vi "Day 20-1.vi"() -> ()   [LabVIEW 2020]
uses:
  Vec2.ctl
panel:
  out "# Lit":i32
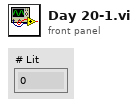
[diagram p1: front panel]
types:
  T1 = typedef "Vec2.ctl" = cluster{"X":i32, "Y":i32}
  T2 = typedef "Puzzle 20-1.ctl" = cluster{"Enhancement":bool[], "Image":map{T1, bool}, "Fill":bool, "Min":T1, "Max":T1}
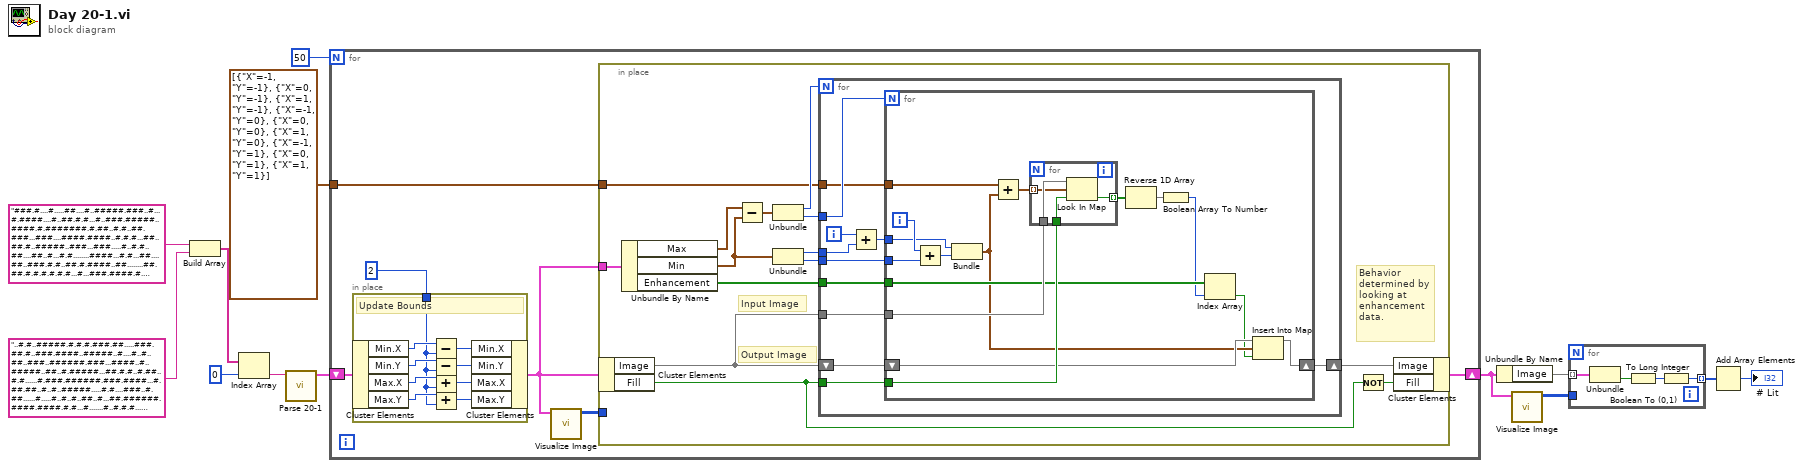
[diagram p0: block diagram]
diagram:
  n1 = Build Array("###.#....#.....##....#..#####.###..#...#.####....#..##.#.#...#..###.#####..####.#.#######.#.##..#.#..##.###...###....####.####..#.#.#...##..##.#..#####..###...###.....#..#.#..##....##..#...#.#........####...#.#...##....##..###.#.#..##.#.####..##........##.##.#.#.#.#.#.#...#...###.####.#.######..#.#.##....#.##.....##.#.#.#.##...#...#.#..#..##.#######.###............####...###.#..#.###.#...#.......#.##.##...##..####.##....#####....#..#...#.#.##.#......#####....#####..#..#.##...#.#....##.##..###....##.#....##.\n\n.......#............#.##...##..#...##.#..####.#..#.##..#.##.##..#.#....#.#####.#.##..#..#..##..#.###\n.#.####.......#....##....#####.##...######.###.##....####..####.#....#..####..#....#.##..##.##..##..\n.###.##.#.##.#......#...##.#.#.##..##..##....##...#####...#####..###......####...###.#.###.##.##.##.\n###.##.....###.##...###..#..##.#.#....####..###.###..###..###.#..#..#..##...#....##..#..####..#...#.\n..#######..#...##..####.#.#.#.##.#.##.######..#.##.#..####.#.##.####.#.#..##.#.....#.#...###.###....\n#.###.#....#.###..#.....##....#..##.....#####..###.#..#.####..#....#......#.#.##.#...#####..#.#.####\n.###.##.##.##..#...#.#.###.#.#####.########.....#####.#.......##...##....#.#.###...#..#...##.#.#.#..\n.###..###....###.###.###.##.###...##.##.....####.#.##.##..#####.#.#.##..##....##.#..#.#..#..#..#.#..\n###.#.....#.##.#..#...###.###..##..##...##..#.#.####.#.###.##.#.###..##..#.##.#.#.#..#####..#.#.#..#\n###.#....#.#...######.##..#.####..##.....#.###.....###...##....###.#######..#......#....####.#..#..#\n..#...#...#.##.#....###.#######....###..###.#####.###.#..#.....#.#.###.#...#.###..##.#.#.##.##.##...\n##...#.....##.#.##.##..#..#...#........##....#.#.#....#..##..####..#....#####.##.##..###.###.####.##\n.#.###.....#...##...#..#..###..#.##..#.##..##.#.##.#.##.#.###...####.#.#...##...####.#....#.#....#.#\n########.#.#.#.....##.##..###.#..#.#####.##.##.##.##.#..#..#.#.###.##########..##...#..###..#.##..#.\n......##.##..##.###.####...###.#..##.#.##.####.####...#######..#..#.###..##...###.###.#.#.#.######.#\n.###.####.#####.#.#.#...##.#.##....#..##.#####.####....#.....##.#.#..##....##..#.#.####...#.##...#.#\n##....######...#..##..#.#####.##.#####..#......#.#.#..#######.#...##.##..##..#..#.###.#.#......##.#.\n.##......#..#...#..##..#.#.###..##.#..###.###.##.##.#...#.#.##.#.###....#####....##...##...####.###.\n####.###....###..###.###......####.#..#####.#......##....#...##..#####....#.#######.##...##.##.##.##\n#....##.####....#####...##......####.#.#.#.##....#.###.#...##.##...#.#.##.#....#..#.##.#.#..#.#..##.\n#.##.#.##..##.#.##...#####.###.#..##.....###...#.##.###....#.###..###.####....###..##.###.#..######.\n..#...##...#...#...#..###..#..#.#......##.#...#...#..#.#..#..#.##.#####...#..##..###...#.###..#....#\n.##...#.#.....#.###...###....#####...##.#.###..##..###.#...######.#####.#..####.#....###.####..#...#\n#.##.##.#.#.#..#.#####.###.###.#.###..#.#.##..####.#.######.#.###.#.##...#..#..#..#.#.#..#.#.#..##..\n#####.####.##.#..##.......#....#...#.#.....#..#.#...#.......##.#######.#.##....#.....##...##...###.#\n##.#...#.#..####.##.###.####..###..###..#...#.######.##.##.#.#.#..###.#.##.#.#.#..#####..###.##....#\n.#.##.#.#......#......###.#.####..#.#..###....#####..###..#.######....##..##.##.##....#..#........#.\n.##.##..#####.....#.###.....#.##....#.....#.#.#..#..#######..#####.....##.###.###.##..##..###...##.#\n#..#.#.#.####..###.#.##.......#.#.#.#.##.#.#.#.#..##.##.##.......#.#.#..#..###...#.##.#.#..#....###.\n.#####.#.##.#..#.#...####...###.####.#.#.....####..#...#.###...#....#.#..####.####...#....#.##.###..\n.....##..#.##.#######....###...##...#.#.##.#..###....#.##..###....##..##.#.###.##..#####........#.##\n##.#.#.#########..##....#..#.##.#...#..#....##..#.###.#.#.#.###.#.....#......##.##....#.....#.#...##\n..##..#..#.##...#.....##.##....##.####....#...###..##...##.#......#...#.....#....##...###.###....#..\n##.#.##.....#.#.##..#......#...####....#.##.#.##..####.##.#.###.#...#..#..##..###..#.###.####.####.#\n.#.#..####.##.#.###..##.#.###..##.##..#...##..#..#.##..####..####..#...###.######....###.#..#####..#\n#.##..##.##...#....##...###..#.##...##....#.....#..##.#.###....#......##.##..###.#..######....##.#..\n#.####.....##.###.##...###.###.#....#.....####.#####......#.#......#..##...##.#....###.##.#....#..#.\n...###..###.#.#.###.#.#.##.####.#.######.#.##..#...#..##.#.#.#.#.............#..#.#.###.....##.###..\n#...###.#.##.####..##...###.##...####.##....######.....######.##.##.#..#.##.##.#......#.###.#.#...##\n####.#.########.##...##.############...###.##...#...######....##.########.##.##..#...##..#.#...##.##\n###.#..#..##.##....#..#..#..##.#.##.##.......##..#...#.###.#.#....##.#.#.##.#####.##.......#.#.#..##\n..#######.####.##...#####.#.####.#...#...#..#..##.###.#########....#..###.##..#.##..##.....###.#..#.\n###.#.#..#.#..###.#.#..#.##...##....#.#..#.......#.###.#.#.#.#####...#...######.##.#....##.#..#.#.#.\n.##....#.#.###...#.#...####..###.#.#.#..##.##.#..##...#...####..#......#####..####..##.##.##...##..#\n...##.##..#.#.....##...#..##.#.#.####..##.........##..##.....#.###.##...##.##..#..#...#..#......####\n......#..#####.....#....##..#####...#.#.##......##....####...#...####.###.#.#.##..#..#...##...###...\n...###....###.####.#....###......#.#...#.##.#..#######..#....#####.##.#####..###....##.##..##....#.#\n##...###.####..#...#.##....#..#.#.#..#.#....#.#...#.##..#..######.....##..#.#.######.#.#....##.#.#.#\n#..##...#..#.##.....####.##.##.#.#.##.#..##..##..#...#####.###.###........#.#.#..#.#.##.#...##..#.#.\n#####..##....#.#..##.#.##..#.###..##..#.#.###.####.#.#..#.....#..##.####..#.####.###..#.....##....##\n.##..###.#.#.#.#.####.#.##...###..#####.####.###.##.###.##.#....#.#.#..#.#.##.#..####...###.####.##.\n#.#.#......#.###.#...###..###...#...#.#..######.###.##.#.####.....#...##.#..##..##.#..##.#.#....#.##\n#...##...##.#...##....######.########....#..#######.#.####....#..##..##.##.#.###.####.####..###.####\n#.##..##...#.####.#.#..####.#.##.#.#...####...####.#.#....####..##...#......#........##........####.\n..##.#..######...#####.#.##.###.##.......#..###..###...#....#..####..#..#..#...##.#.##.####.#.##.#..\n#..#...###..#..#.#...###.#..#.#...#.....##..#.#...#####...##....##.......####.##..####..##.#..######\n.##.####..###..##.#.####.###.##...##..###.#.#.##...##.....#..#..#.####..###...##...#######.....##.#.\n.####.#.#.##...##...###.....####.##..####....##....#...##.##...##.####.###.##...#####..#...#.#...#..\n....#.#...#..#.#.#....####.##..#.#....#........#...####..###..###.###...#..###.#..#.##.#..#...#.####\n#..#..##..##.#...#####...#.......#..##..###.#.#.####..###.#...##......##.##.#..#.#.##.#..##.#.#...#.\n.#####...#.##.###.#.##..###.##.#.#...##..#.#...###.....##.#.##.#..#..####...#.######....#..#.##..#..\n#.#...#.....#.....######.##.##.##.##.#.#..#..#.#.####..#...#####.##.####..###.##.#.#.#.#..#.#...####\n##.##.#.#...##.#.###.#####.#...##.........#......#.##.....#.......##....#.#.##..#.#..#.#..##..#.###.\n....#.#.##.###.##..##.#..#.##.#..#.######.###.##..#..#.#...###.#........###.###.##..####.#...###..#.\n#####..####.#.###..#####...#.......#.##.#.....#.###.####.......##.#.#.##.#...#....#....#....##...##.\n.##.#..####...##...##.....##..#.####.#...#..##..#....####.#..#..#.#..#...#.#.#.##.####..######..#.#.\n#.#.##.##.#.....#...#..#...#.#.#..#.#.#####..#.##..#.##.#......##.#..#.#.#...#...####.#.#.#.#....#..\n.##..###.##..##...#..##...#..#......#.#####.####.####.#.......##.#.#..#..#.#.##.#..#..###.#.#..##..#\n#..##...#........##..#...###########.#.###...##.##...##.#.###...####..########..#...##..####..###...\n.#.#..###.#.##.#.#..#######......####.#....#####...##...#.###.##....#####.#...#######.######..######\n.#.###..###.##...#...###.########...#.#.#.#..#...#..#.#.....####..#...####......#.#...##.#.###..##.#\n#.###.###...#..#####.###.#...###..#..#..###.#..#..###.#..##.####..#####..#....#....##.##.#..#.####.#\n..#.###.#.#.#.#...####.#.##.#...#.##...#.###.##.#.#######.#####.##..####....###.###.##.#.##....##.##\n#..#.....#..#.##.#....#.####..#.##..####.#..#.#.###..##..#..#..##.####........#..#....#.#.#.###.##..\n#.##.#.#..##.#####...##.#...#..#...#.#.##.#..##.....##.##.#.#.#.###......#.###.###..###.###..#######\n##.###.###...#..##.....#######..##.#.##..#.#.....###.#....####.####.#..##.#..#..#..##.....#..###..##\n#....#..#.#.#..#.#....#.##.#.#.#.###.###.###.##..##.####..####.#.#....#.#######..###.#.....####.#..#\n###.....#.#####..###.#.#....#.....#.###....##..###.#..#.#.#...###.##....#....#..#......#..#....#..#.\n.#.#.#.#####........#.#######...#.####...#...#.###..#....#.#.###.##.....##.#.##..#.#.....#.#..##..##\n...###..#....#.###.#.#.#..##.##.....##.##...#.#........#.#.#####.#...####.#...##..##......#####.###.\n##.###..#.#...#......#######.#..##....###.#.##.#..###.#..###.#...#..######..........##.#.#.#..#..##.\n#..###.#...##..#######..#..#.###..#.###.##.######.##.###.##..#######.#..###.##.##...###....##..#.#.#\n#.#....#..#.###.#.##...#####.##....#...#.##.#..#.##..#...#...##.#..#..#.#.#..#####..##.###....#.#.##\n###...#.#.#..####.....##.#.##.##..#.####...###....###.#.##.########..#####.##.##.#..#....###..###.##\n##.###...#.#.#.#.##...##.#.##.#.#..#.#.#.###.##.#.##.##....########.#..#####..##.#.#.#..#####.#..###\n##..##.##.###.#######.##.......#.#.##.###..##...#...##...#####.#....#.#.#...#.#..#.#.#..####.###.#.#\n###..#.#..#..#..####.#.#.####..#....######...####..######.##.##..#####....####...##########..#####.#\n...#####.#.##....##.##....#...##...##.#.#.#.#.......#.##.#...####.##..####.....#...##..##.#...##...#\n#####.#.###..#..###.#..#..##..##.#.#.#.#..#...###...#.###.###.###..#.#.##.#####...#.#.##.#....#####.\n###.#..###.#.####.#.#..#.##.##.#.#.##......##.####..#...#....##..#....#.#..#..##...###...##.##.#.#..\n..#.#..#...##.#....###.##...#...##.##..###..#.#.#.......##.#.#..#.##.#......#.#..#..#...#...#.#.#.##\n#.#.#.#..###.##.#.#####.###.#.#..###....###...###....#.#..#.......##.#.###..##..#...###.#.##....#..#\n.#..##......#.#.....##.#...##....####....##.####..#....#...##.######.#..#.#.#....#.#######.....####.\n..#..###....##.##..##..#.#..####..##...#.####..........##.#.#.#..##..#..#.##....###.####.....#..##.#\n....#.#.....#.#..#....#..#.###.####..#..##.####....##....#.#..#.#.####.##.......##.##.###.#.##..#.#.\n..###.##....#.##......####..###..#..##.########.###.##...###.#.....#...###.#..#..#.#....#..#.######.\n.##.#.........#..#.#..#.#.##.####.#..##...#.###....#..#...##..##.#..#..####.#...#...####.....##...##\n##..#.#.##.##.#...######..##.##.#.#.#.###..#.#.#....###......##...#.#....#...##.########.##..####.##\n.#......##.###...##..##..###.####.#....##.#.#.#....##.#....##...######.....##..##....#.###..#..#.##.\n#...#...#.......#.#.#####.#..###..#..#...###...###..#.#.......###.#..##.#####...##.#####...#.#.####.", "..#.#..#####.#.#.#.###.##.....###.##.#..###.####..#####..#....#..#..##..###..######.###...####..#..#####..##..#.#####...##.#.#..#.##..#.#......#.###.######.###.####...#.##.##..#..#..#####.....#.#....###..#.##......#.....#..#..#..##..#...##.######.####.####.#.#...#.......#..#.#.#...####.##.#......#..#...##.#.##..#...##.#.##..###.#......#.#.......#.#.#.####.###.##...#.....####.#..#..#.##.#....##..#.####....##...##..#...#......#.#.......#.......##..####..#...#.#.#...##..#.#..###..#####........#..####......#..#\n\n#..#.\n#....\n##..#\n..#..\n..###") -> (w11:string[])
  n2 = Index Array(array=w11, index=0) -> (element=w9:string)
  n3 = call "Parse 20-1.vi"("String"=w9) -> ("Puzzle"=w8:T2)  [unwired: 10 in]
  n4 = for {
    N: 50 -> [_]
    shift-right: [w18] -> w2
    shift-left: w8 -> [w19]
    tunnel: T1[] [{"X"=-1, "Y"=-1}, {"X"=0, "Y"=-1}, {"X"=1, "Y"=-1}, {"X"=-1, "Y"=0}, {"X"=0, "Y"=0}, {"X"=1, "Y"=0}, {"X"=-1, "Y"=1}, {"X"=0, "Y"=1}, {"X"=1, "Y"=1}] -> [w17]
    n5 = in-place {
      in-place-border: 2 -> [w65]
      # "Update Bounds"
      n6 = in-place-cluster #1(w19) -> ("Min.X"=w73:i32, "Min.Y"=w70:i32, "Max.X"=w67:i32, "Max.Y"=w66:i32)
      n7 = Subtract(x=w73, y=w65) -> (x-y=w72:i32)
      n8 = Subtract(x=w70, y=w65) -> (x-y=w71:i32)
      n9 = Add(x=w67, y=w65) -> (x+y=w69:i32)
      n10 = Add(x=w66, y=w65) -> (x+y=w68:i32)
      n11 = in-place-cluster #1("Min.X"=w72, "Min.Y"=w71, "Max.X"=w69, "Max.Y"=w68) -> (w16:T2)
    }
    n12 = call "Visualize Image.vi"("Puzzle 20-1"=w16) -> ("Image"=w15:i16[][])  [unwired: 10 in]
    n13 = in-place {
      in-place-border: w16 -> [w33]
      in-place-border: w17 -> [w22]
      in-place-border: w15 -> [_]
      # "Input Image"
      # "Output Image"
      # "Behavior determined by looking at enhancement data."
      n14 = in-place-cluster #2(w16) -> ("Image"=w20:map{T1, bool}, "Fill"=w21:bool)
      n15 = Unbundle By Name(w33) -> ("Max"=w32:T1, "Min"=w29:T1, "Enhancement"=w25:bool[])
      n16 = Subtract(x=w32, y=w29) -> (x-y=w31:T1)
      n17 = Unbundle(w31) -> ("X"=w30:i32, "Y"=w28:i32)
      n18 = Unbundle(w29) -> ("X"=w27:i32, "Y"=w26:i32)
      n19 = for {
        N: w30 -> [_]
        tunnel: w28 -> [w44]
        tunnel: w27 -> [w43]
        tunnel: w26 -> [w40]
        tunnel: w25 -> [w39]
        shift-right: [w37] -> w24
        shift-left: w20 -> [w38]
        tunnel: w22 -> [w35]
        tunnel: w20 -> [w34]
        tunnel: w21 -> [w36]
        i -> [w42]
        n20 = Add(x=w42, y=w43) -> (x+y=w41:i32)
        n21 = for {
          N: w44 -> [_]
          tunnel: w41 -> [w58]
          tunnel: w40 -> [w60]
          tunnel: w39 -> [w51]
          shift-right: [w46] -> w37
          shift-left: w38 -> [w49]
          tunnel: w35 -> [w56]
          tunnel: w34 -> [w54]
          tunnel: w36 -> [w53]
          i -> [w59]
          n22 = Add(x=w59, y=w60) -> (x+y=w57:i32)
          n23 = Bundle(w58, w57) -> (w48:cluster{i32, i32})  [unwired: 1 in]
          n24 = Add(x=w56, y=w48) -> (x+y=w55:T1[])
          n25 = for {
            tunnel: w55 -> [w62] mode=indexing
            tunnel: w54 -> [w64]
            tunnel: w53 -> [w63]
            tunnel: [w61] -> w52 mode=indexing
            n26 = Look In Map(map=w64, key=w62, default value=w63) -> (value=w61:bool)  [unwired: 1 out]
          }
          n27 = Reverse 1D Array(array=w52) -> (reversed array=w45:bool[])
          n28 = Boolean Array To Number(Boolean array=w45) -> (number=w50:u32)
          n29 = Index Array(array=w51, index=w50) -> (element=w47:bool)
          n30 = Insert Into Map(map in=w49, key=w48, value=w47) -> (map out=w46:map{T1, bool})  [unwired: 2 out]
        }
      }
      n31 = Not(x=w21) -> (.not. x?=w23:bool)
      n32 = in-place-cluster #2("Image"=w24, "Fill"=w23) -> (w18:T2)
    }
  }
  n33 = Unbundle By Name(w2) -> ("Image"=w5:map{T1, bool})
  n34 = call "Visualize Image.vi"("Puzzle 20-1"=w2) -> ("Image"=w1:i16[][])  [unwired: 10 in]
  n35 = for {
    tunnel: w5 -> [w77] mode=indexing
    tunnel: [w74] -> w4 mode=indexing
    tunnel: w1 -> [_]
    n36 = Unbundle(w77) -> ("value"=w76:bool)  [unwired: 1 out]
    n37 = Boolean To (0,1)(Boolean=w76) -> (0, 1=w75:i16)
    n38 = To Long Integer(number=w75) -> (32bit integer=w74:i32)
  }
  n39 = Add Array Elements(numeric array=w4) -> (sum=→"# Lit":i32)
